vi "[GV]_IMU pitch.vi"() -> ()   [LabVIEW 2016]
panel:
  in  "IMU pitch":dbl
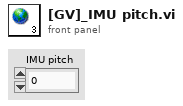
[diagram p1: front panel]
diagram:
